vi "JGP1.vi"() -> ()   [LabVIEW 2019]
doc: "Force Calculator using two masses and gravity \nForce analysis for paired strain Sensors\nJuan Gamez\nP3600\nCSUSB Physics"
panel:
  out "F right (N)":dbl=15.696000000000002
  out "F left (N)":dbl=23.544
  out "Y (Nm)":dbl caption="Applied Torque Y (Nm)"
  out "X (N)":dbl=39.24 caption="Applied Force X (N)"
  in  "B (m)":dbl=3.0 format="%_3g"
  in  "A (m)":dbl=2.0 format="%_3g"
  in  "D (m)":dbl=3.0 format="%_3g"
  in  "g (m/s^2)":dbl=9.81 caption="gravity (m/s^2)" format="%_3g"
  in  "m right (Kg)":dbl=2.0 format="%_3g"
  in  "m left (Kg)":dbl=2.0 format="%_3g"
  # "Resultant Force Analysis for Paired Strain Sensors"
  # "Masses"
  # "Problem 1 \nJG\nP3600\nCSUSB Physics"
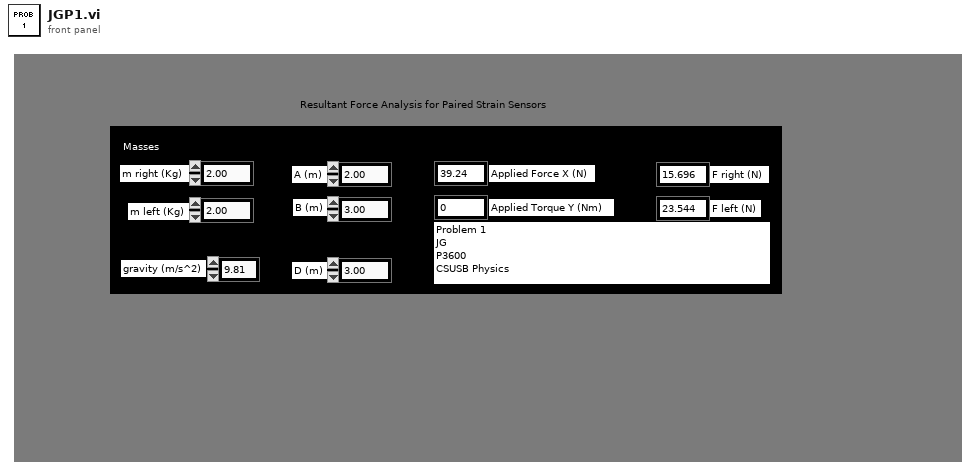
[diagram p1: front panel]
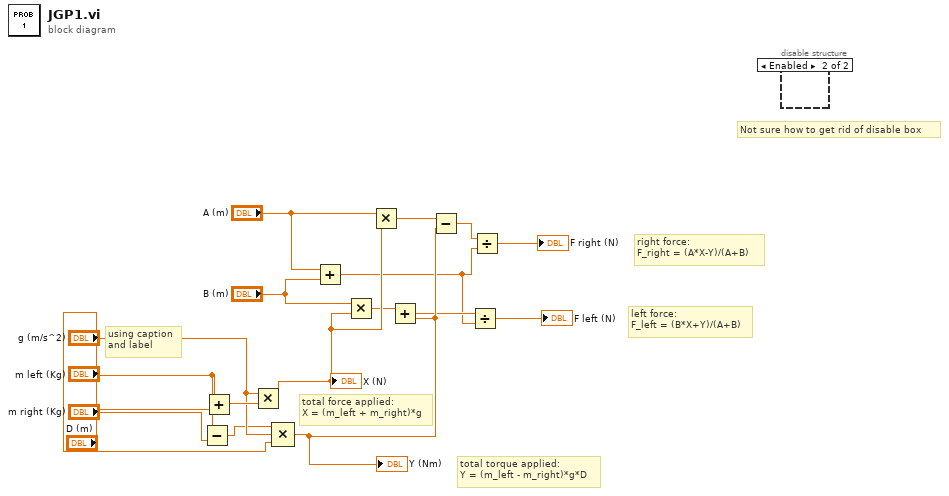
[diagram p0: block diagram]
diagram:
  # "Not sure how to get rid of disable box"
  # "left force:\nF_left = (B*X+Y)/(A+B)"
  # "right force:\nF_right = (A*X-Y)/(A+B)"
  # "total torque applied:\nY = (m_left - m_right)*g*D"
  # "total force applied:\nX = (m_left + m_right)*g"
  # "using caption\nand label"
  n1 = Subtract(x="m left (Kg)", y="m right (Kg)") -> (x-y=w13:dbl)
  n2 = Add(x="m left (Kg)", y="m right (Kg)") -> (x+y=w17:dbl)
  n3 = Multiply(x="g (m/s^2)", y=w17) -> (x*y=w6:dbl)
  "X (N)" <- w6
  n4 = Compound Arithmetic op=MULTIPLY(w13, "g (m/s^2)", "D (m)") -> (w4:dbl)
  "Y (Nm)" <- w4
  n5 = Add(x="A (m)", y="B (m)") -> (x+y=w2:dbl)
  n6 = Multiply(x="B (m)", y=w6) -> (x*y=w5:dbl)
  n7 = Multiply(x="A (m)", y=w6) -> (x*y=w11:dbl)
  n8 = Add(x=w5, y=w4) -> (x+y=w3:dbl)
  n9 = Subtract(x=w11, y=w4) -> (x-y=w9:dbl)
  n10 = Divide(x=w3, y=w2) -> (x/y=→"F left (N)":dbl)
  n11 = Divide(x=w9, y=w2) -> (x/y=→"F right (N)":dbl)
  n12 = disable-structure shown="Enabled" {
    frame Disabled {
    }
    frame Enabled {
    }
  }
